vi "Load Classes Names and Dict.vi"(8 "error in (no error)":errorcluster, 9 "Class Rerative Paths Path":path, 10 "Reference Class Path":path) -> (0 "error out":errorcluster, 2 "Classes Map":T1)   [LabVIEW 2023, in "Class Loader.lvlib" / "Class Loader.lvclass"]
uses:
  Class Loader.lvclass
  Classes Map.ctl
  65303d96-c5e3-48a2-9982-32b5e917b9e9.vi
  65303d96-c5e3-48a2-9982-32b5e917b9e9.vi/b0178052-0c48-4c9a-874f-40b592e34ac5.vi
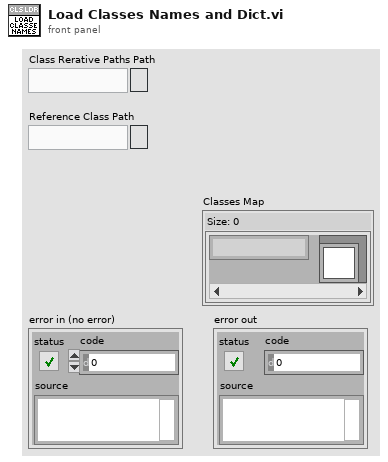
[diagram p1: front panel]
types:
  T1 = typedef "Class Loader.lvlib/Class Loader.lvclass/Classes Map.ctl" = map{string, refnum<class>}
  T2 = typedef "Class Loader.lvlib/Class Loader.lvclass/Class Details.ctl" = cluster{"Class Name":string, "Class":refnum<class>}
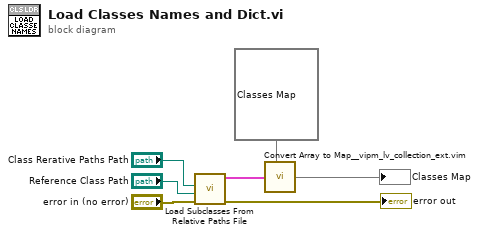
[diagram p0: block diagram]
diagram:
  n1 = call "Load Subclasses From Relative Paths File.vi"("error in"="error in (no error)", "Reference Class Path"="Reference Class Path", "Class Relative Paths Path"="Class Rerative Paths Path") -> ("error out"=→"error out":errorcluster, "Class Details Array"=w2:T2[])  [unwired: 5 in, 2 out]
  n2 = call "Convert Array to Map__vipm_lv_collection_ext.vim"("map type (optional)"=T1 {} ("map"), "array"=w2) -> ("map"=→"Classes Map":T1)  [unwired: 5 in]
